vi "Cleanup Session.vi"(8 "error in":errorcluster, 11 "Plugin in":refnum<class "Digital Output Handler.lvclass">) -> (0 "error out":errorcluster, 3 "Plugin out":refnum<class "Digital Output Handler.lvclass">)   [LabVIEW 2023, in "Digital Output Handler.lvlib" / "Digital Output Handler.lvclass"]
uses:
  Digital Output Handler.lvclass
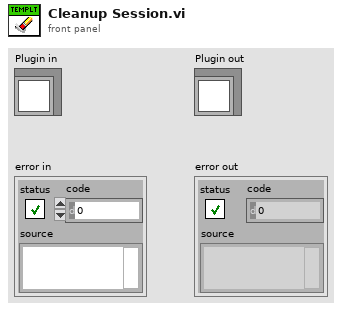
[diagram p1: front panel]
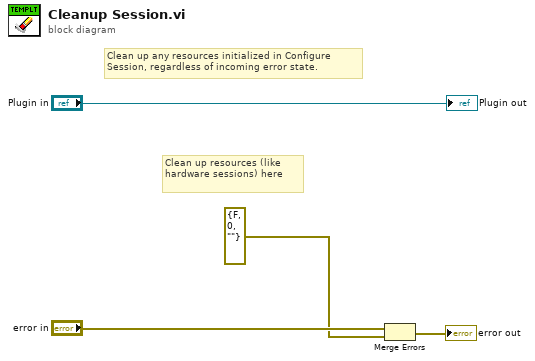
[diagram p0: block diagram]
diagram:
  # "Clean up resources (like hardware sessions) here"
  # "Clean up any resources initialized in Configure Session, regardless of incoming error state."
  n1 = Merge Errors("error in", errorcluster {"status"=FALSE, "code"=0, "source"=""} ("error in")) -> (→"error out":errorcluster)
  "Plugin out" <- "Plugin in"
